vi "Initialise notifiers and events.vi"(8 "error in (no error)":errorcluster, 11 "SubscriptionDetails JSON in":refnum<class "SubscriptionDetails JSON.lvclass">) -> (0 "error out":errorcluster, 3 "SubscriptionDetails JSON out":refnum<class "SubscriptionDetails JSON.lvclass">)   [LabVIEW 2020, in "wamplv.lvlib" / "SubscriptionDetails JSON.lvclass"]
uses:
  SubscriptionDetails JSON.lvclass
  SubscriptionDetails JSON.lvclass/SubscriptionDetails JSON.ctl
  WAMP Client/Private/TypeDef/EVENT payload (JSON).ctl
  wamplv.lvlib
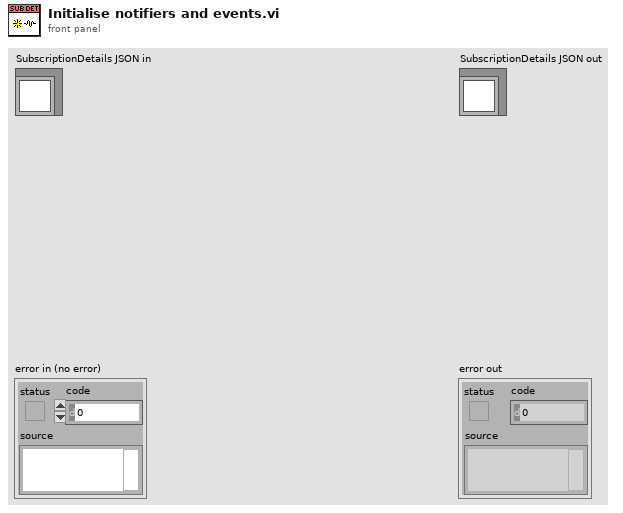
[diagram p1: front panel]
types:
  T1 = typedef "wamplv.lvlib/EVENT payload (JSON).ctl" = cluster{"Publication ID":u64, "Topic":string, "Arguments Payload":string, "ArgumentKw Payload":string, "Details":string}
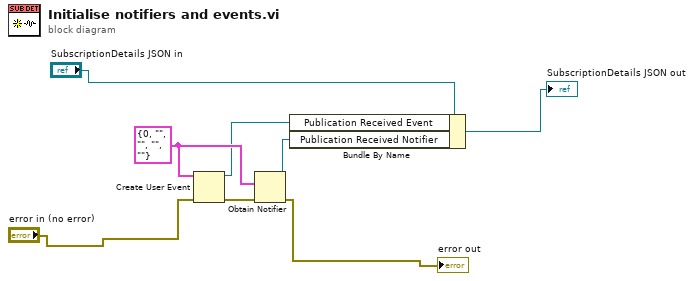
[diagram p0: block diagram]
diagram:
  w8 = T1 {"Publication ID"=0, "Topic"="", "Arguments Payload"="", "ArgumentKw Payload"="", "Details"=""} ("Cluster")
  n1 = Create User Event(user event datatype=w8, error in="error in (no error)") -> (user event=w6:refnum<user-event>, error out=w7:errorcluster)
  n2 = Obtain Notifier(notification data type=w8, error in (no error)=w7) -> (notifier out=w5:refnum<notifier>, error out=→"error out":errorcluster)  [unwired: 2 in, 1 out]
  n3 = Bundle By Name(cluster="SubscriptionDetails JSON in", "Publication Received Event"=w6, "Publication Received Notifier"=w5) -> (→"SubscriptionDetails JSON out":refnum<class "SubscriptionDetails JSON.lvclass">)
